vi "Create_Video_Catalogue.vi"() -> ()   [LabVIEW 2015]
panel:
  out "File number":i32=4
  in  "stop":bool
  out "Copy From":path=path "Z:/2015/EnFlo_Tunnel/Paul_Hayden/Raw_Measurements/Raw_Meas_11-2015/Flow_Vis_Res_4_xls/Flow_Vis_Res_4_8.xls"
  in  "Destination Folder":path=path "Z:/2015/EnFlo_Tunnel/Paul_Hayden/Results_Post_Processed/Diplos/2015/Flow_Vis/Video Catalogue2"
  in  "Video Name":string="Video_name::"
  in  "Raw Data Filename":string="Raw Data File::"
  out "Ch names Out":string[](array[string])=["Case::", "Wind Direction Deg::", "Plane::", "Plane Location::", "Source::", "Laser Power (mW)::", "Uref::", "Source Q l/min::", "Source Type::", "File::", "Raw Data File::", "Seconds::", "Video_name::"]
  in  "Run Log folder":path=path "Z:/2015/EnFlo_Tunnel/Paul_Hayden/Results_Post_Processed/Diplos/2015/Flow_Vis/Flow_Vis Run_Log.xls"
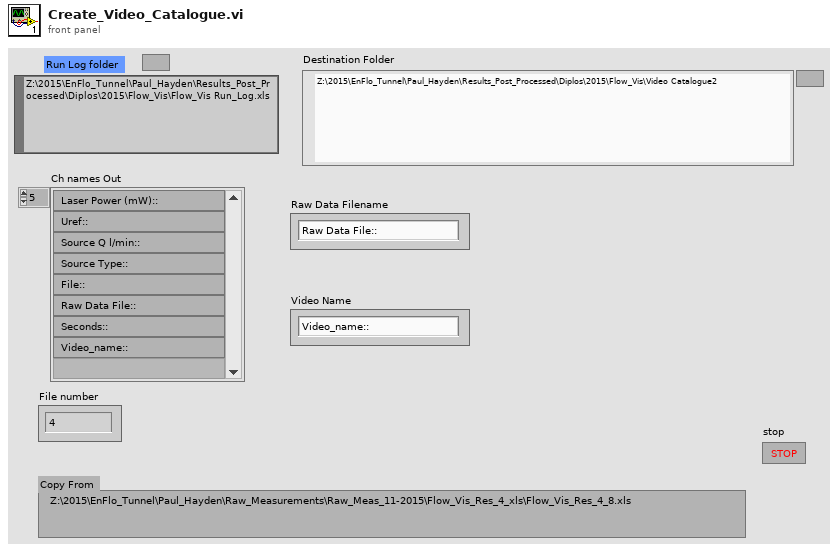
[diagram p1: front panel]
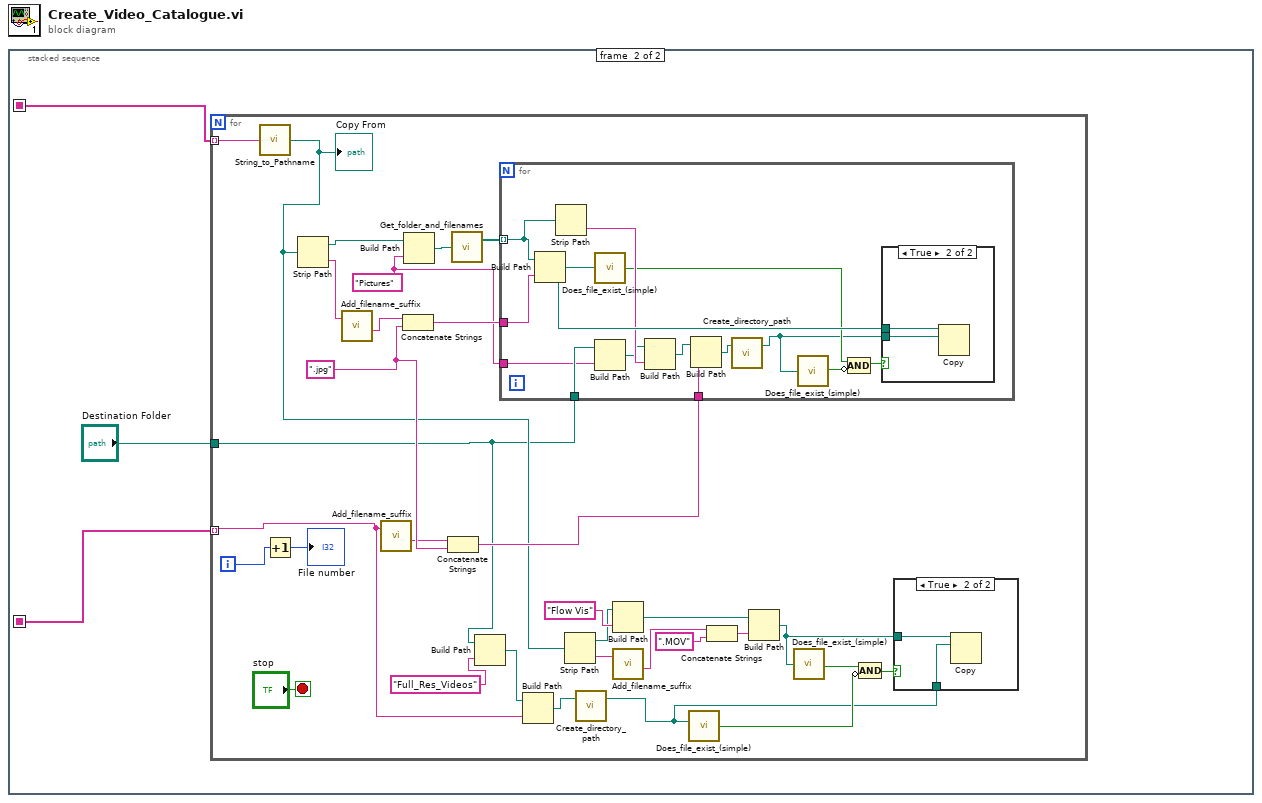
[diagram p0: block diagram]
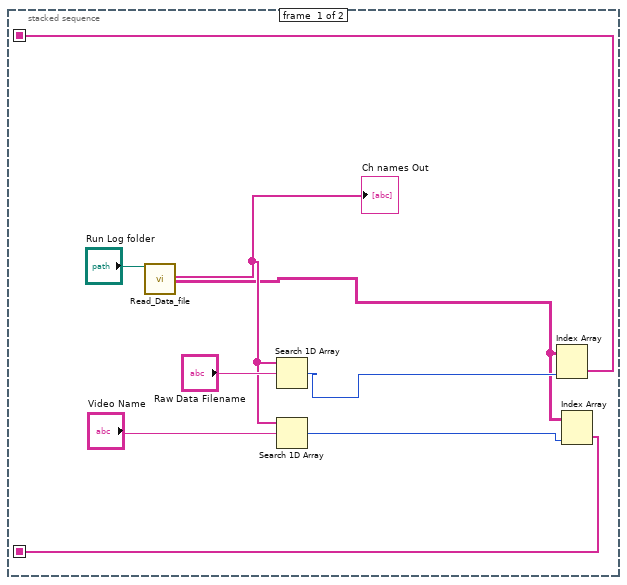
[diagram p2: hidden frame]
diagram:
  n1 = stacked-sequence {
    seq-local: [w2 _] -> [_ w12]
    seq-local: [w1 _] -> [_ w10]
    frame #0 {
      n2 = call "Read_Data_file.vi"("Results file"="Run Log folder") -> ("Ch names Out"=w6:string[], "Channel Values Out"=w3:string[][])  [unwired: 9 in, 8 out]
      "Ch names Out" <- w6
      n3 = Search 1D Array(1D array=w6, element="Raw Data Filename") -> (index of element=w7:i32)  [unwired: 1 in]
      n4 = Search 1D Array(1D array=w6, element="Video Name") -> (index of element=w4:i32)  [unwired: 1 in]
      n5 = Index Array(array=w3, index (col)=w7) -> (element=w2:string[])  [unwired: 1 in]
      n6 = Index Array(array=w3, index (col)=w4) -> (element=w1:string[])  [unwired: 1 in]
    }
    frame #1 {
      n7 = for {
        tunnel: w12 -> [w44] mode=indexing
        tunnel: "Destination Folder" -> [w16]
        tunnel: w10 -> [w21] mode=indexing
        i -> [w41]
        stop <- "stop" stop-if-true
        w35 = ".jpg" ("x")
        w36 = "Pictures" ("name or relative path")
        n8 = call "String_to_Pathname.vi"("Input String"=w44) -> ("path"=w23:path)
        "Copy From" <- w23
        n9 = Increment(x=w41) -> (x+1=→"File number":i32)
        n10 = Strip Path(path=w23) -> (stripped path=w31:path, name=w43:string)
        n11 = call "Add_filename_suffix.vi"("Filename"=w43) -> ("Base name"=w32:string)  [unwired: 1 in, 3 out]
        n12 = call "Add_filename_suffix.vi"("Filename"=w21) -> ("Base name"=w34:string)  [unwired: 1 in, 3 out]
        n13 = Concatenate Strings(w32, w35) -> (w37:string)
        n14 = Build Path(base path=w31, name or relative path=w36) -> (appended path=w39:path)
        n15 = Concatenate Strings(w34, w35) -> (w33:string)
        n16 = call "Get_folder_and_filenames.vi"("file path (dialog if empty)"=w39) -> ("Folders"=w38:path[])  [unwired: 1 out]
        n17 = Build Path(base path=w16, name or relative path="Full_Res_Videos") -> (appended path=w15:path)
        n18 = for {
          tunnel: w16 -> [w60]
          tunnel: w38 -> [w56] mode=indexing
          tunnel: w37 -> [w59]
          tunnel: w36 -> [w58]
          tunnel: w33 -> [w54]
          n19 = Build Path(base path=w56, name or relative path=w59) -> (appended path=w57:path)
          n20 = Strip Path(path=w56) -> (name=w55:string)  [unwired: 1 out]
          n21 = call "Does_file_exist_(simple).vi"("Pathname"=w57) -> ("exists?"=w49:bool)
          n22 = Build Path(base path=w60, name or relative path=w58) -> (appended path=w53:path)
          n23 = Build Path(base path=w53, name or relative path=w55) -> (appended path=w51:path)
          n24 = Build Path(base path=w51, name or relative path=w54) -> (appended path=w52:path)
          n25 = call "Create_directory_path.vi"("Path name"=w52) -> ("Path name Out"=w47:path)  [unwired: 1 in, 1 out]
          n26 = call "Does_file_exist_(simple).vi"("Pathname"=w47) -> ("exists?"=w50:bool)
          n27 = Compound Arithmetic op=AND(w49, invert w50) -> (w48:bool)
          n28 = case shown="True" w48 {
            tunnel: w57 -> [_ w62]
            tunnel: w47 -> [_ w61]
            frame False {
            }
            frame True {
              n29 = Copy(10:w61, 11:w62) -> ()  [unwired: 3 in, 3 out]
            }
          }
        }
        n30 = Build Path(base path=w15, name or relative path=w21) -> (appended path=w14:path)
        n31 = Strip Path(path=w23) -> (stripped path=w24:path, name=w29:string)
        n32 = call "Create_directory_path.vi"("Path name"=w14) -> ("Path name Out"=w13:path)  [unwired: 1 in, 1 out]
        n33 = Build Path(base path=w24, name or relative path="Flow Vis") -> (appended path=w28:path)
        n34 = call "Add_filename_suffix.vi"("Filename"=w29) -> ("Base name"=w27:string)  [unwired: 1 in, 3 out]
        n35 = call "Does_file_exist_(simple).vi"("Pathname"=w13) -> ("exists?"=w20:bool)
        n36 = Concatenate Strings(w27, ".MOV" ("x")) -> (w25:string)
        n37 = Build Path(base path=w28, name or relative path=w25) -> (appended path=w18:path)
        n38 = call "Does_file_exist_(simple).vi"("Pathname"=w18) -> ("exists?"=w19:bool)
        n39 = Compound Arithmetic op=AND(w19, invert w20) -> (w22:bool)
        n40 = case shown="True" w22 {
          tunnel: w13 -> [_ w46]
          tunnel: w18 -> [_ w45]
          frame False {
          }
          frame True {
            n41 = Copy(10:w46, 11:w45) -> ()  [unwired: 3 in, 3 out]
          }
        }
      }
    }
  }
